vi "Interface.RT FIFO.Write.vi"   [LabVIEW 2017, in "DSF Core.lvlib" / "Interface.lvclass"]
uses:
  Interface.lvclass
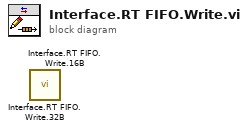
[diagram p0: block diagram]
diagram:
  n1 = call "Interface.RT FIFO.Write.32B.vi"() -> ()  [unwired: 9 in, 3 out]
  n2 = call "Interface.RT FIFO.Write.16B.vi"() -> ()  [unwired: 9 in, 3 out]
